vi "MSC ROI Type to IMAQ ROI Type.vi"(0 "MSC ROI Type":T1 items=["Point", "Line", "Rectangle", "Oval", "Freehand / Polygon"], 11 "error in (no error)":errorcluster) -> (4 "IMAQ ROI Type":u32(ring)=4 items=["No Selection", "Point", "Line", "Rectangle", "Oval", "Polygon", "Freehand Region", "Annulus", "Unused2", "Unused3", "Broken Line", "Freehand Line", "Rotated Rectangle"], 15 "error out":errorcluster)   [LabVIEW 2014]
doc: "Conversion from MSC Picture type to IMAQ type"
uses:
  MSC Image_class/controls/ROI Type.ctl
  MSC Image_class/MSC Image.lvclass
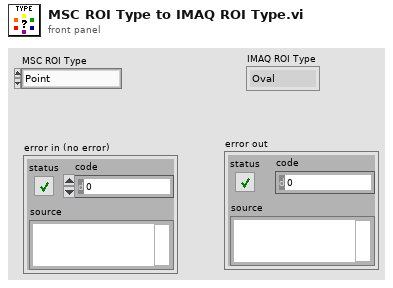
[diagram p1: front panel]
types:
  T1 = typedef "MSC Image.lvclass/ROI Type.ctl" = u16
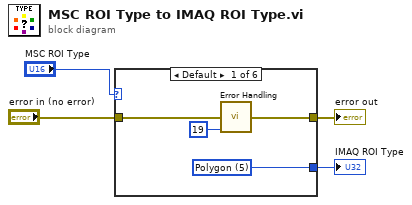
[diagram p0: block diagram]
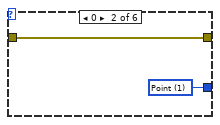
[diagram p2: hidden frame]
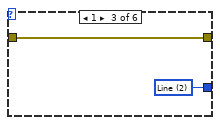
[diagram p3: hidden frame]
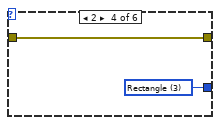
[diagram p4: hidden frame]
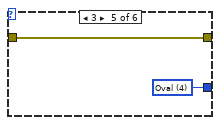
[diagram p5: hidden frame]
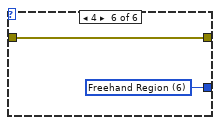
[diagram p6: hidden frame]
diagram:
  n1 = case shown="Default" "MSC ROI Type" {
    tunnel: "error in (no error)" -> [w5 w10 w12 w14 w16 w18]
    tunnel: [w6 w10 w12 w14 w16 w18] -> w3
    tunnel: [w8 w9 w11 w13 w15 w17] -> w1
    frame Default {
      w8 = u32 5 items=["No Selection", "Point", "Line", "Rectangle", "Oval", "Polygon", "Freehand Region", "Annulus", "Unused2", "Unused3", "Broken Line", "Freehand Line", "Rotated Rectangle"] ("Type")
      n2 = call "Error Handling.vi"("error in (no error)"=w5, "return type"=19 ("code")) -> ("error out"=w6:errorcluster)  [unwired: 12 in, 1 out]
    }
    frame 0 {
      w9 = u32 1 items=["No Selection", "Point", "Line", "Rectangle", "Oval", "Polygon", "Freehand Region", "Annulus", "Unused2", "Unused3", "Broken Line", "Freehand Line", "Rotated Rectangle"] ("Type")
    }
    frame 1 {
      w11 = u32 2 items=["No Selection", "Point", "Line", "Rectangle", "Oval", "Polygon", "Freehand Region", "Annulus", "Unused2", "Unused3", "Broken Line", "Freehand Line", "Rotated Rectangle"] ("Type")
    }
    frame 2 {
      w13 = u32 3 items=["No Selection", "Point", "Line", "Rectangle", "Oval", "Polygon", "Freehand Region", "Annulus", "Unused2", "Unused3", "Broken Line", "Freehand Line", "Rotated Rectangle"] ("Type")
    }
    frame 3 {
      w15 = u32 4 items=["No Selection", "Point", "Line", "Rectangle", "Oval", "Polygon", "Freehand Region", "Annulus", "Unused2", "Unused3", "Broken Line", "Freehand Line", "Rotated Rectangle"] ("Type")
    }
    frame 4 {
      w17 = u32 6 items=["No Selection", "Point", "Line", "Rectangle", "Oval", "Polygon", "Freehand Region", "Annulus", "Unused2", "Unused3", "Broken Line", "Freehand Line", "Rotated Rectangle"] ("Type")
    }
  }
  "error out" <- w3
  "IMAQ ROI Type" <- w1
